vi "write_binary_file_with_text_api.vi"   [LabVIEW 2021]
types:
  T1 = enum16{"open", "replace", "create", "open or create", "replace or create", "replace or create with confirmation"}
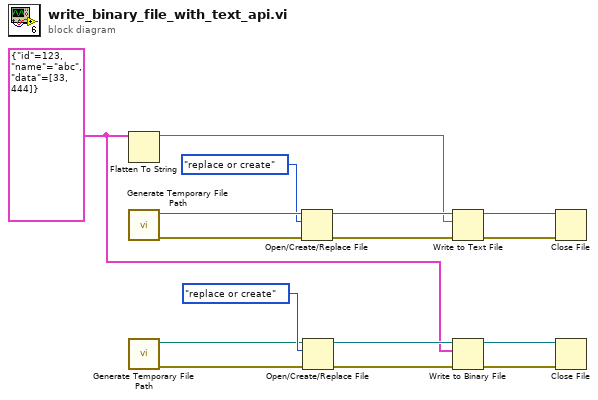
[diagram p0: block diagram]
diagram:
  w5 = cluster{"id":i32, "name":string, "data":i32[]} {"id"=123, "name"="abc", "data"=[33, 444]}
  n1 = Flatten To String(anything=w5) -> (data string=w11:string)  [unwired: 3 in, 2 out]
  n2 = call <vilib>:"Generate Temporary File Path.vi"() -> ("error out"=w15:errorcluster, "Unique Temporary File Path"=w16:path)  [unwired: 10 in]
  n3 = call <vilib>:"Generate Temporary File Path.vi"() -> ("error out"=w7:errorcluster, "Unique Temporary File Path"=w6:path)  [unwired: 10 in]
  n4 = Open/Create/Replace File(file path (use dialog)=w16, error in=w15, operation (0:open)=T1."replace or create") -> (refnum out=w13:refnum<file>, error out=w12:errorcluster)  [unwired: 3 in, 1 out]
  n5 = Open/Create/Replace File(file path (use dialog)=w6, error in=w7, operation (0:open)=T1."replace or create") -> (refnum out=w9:refnum<file>, error out=w10:errorcluster)  [unwired: 3 in, 1 out]
  n6 = Write to Text File(file (use dialog)=w13, text=w11, error in=w12) -> (refnum out=w4:refnum<file>, error out=w3:errorcluster)  [unwired: 1 in, 1 out]
  n7 = Write to Binary File(file (use dialog)=w9, data=w5, error in=w10) -> (refnum out=w2:refnum<file>, error out=w1:errorcluster)  [unwired: 3 in, 1 out]
  n8 = Close File(refnum=w4, error in=w3) -> ()  [unwired: 2 out]
  n9 = Close File(refnum=w2, error in=w1) -> ()  [unwired: 2 out]
